vi "Unpack Control Drag Source Update.vi"(0 "ControlDragSourceUpdateMsg In":refnum<class "ControlDragSourceUpdateMsg.lvclass">) -> (4 "Ctl Refnum":refnum<vi>, 6 "Control Label":string, 8 "Time":u32, 10 "Result":enum16{"Drop Cancel", "Drop Move", "Drop Copy"}(ring))   [LabVIEW 2017, in "ActorEvents.lvlib" / "ControlDragSourceUpdateMsg.lvclass"]
doc: "<License>\nCopyright © 2017 Composed Systems, LLC | All rights reserved\nwww.composed.io\n\nAuthor: Ethan Stern <ethan.stern@composed.io>\n\nThis software is provided \"AS IS\" WITHOUT WARRANTIES, either express or implied, AND IS FOR EDUCATIONAL PURPOSES ONLY.\n</License>"
uses:
  ControlDragSourceUpdateMsg.lvclass
  ControlDragSourceUpdateMsg.lvclass/ControlDragSourceUpdateMsg.ctl
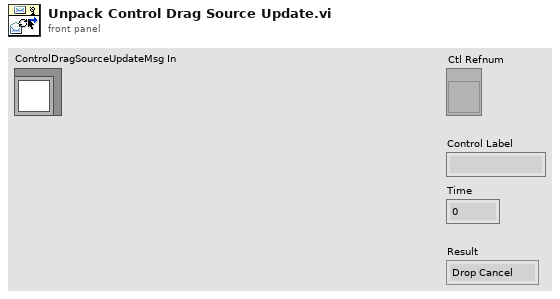
[diagram p1: front panel]
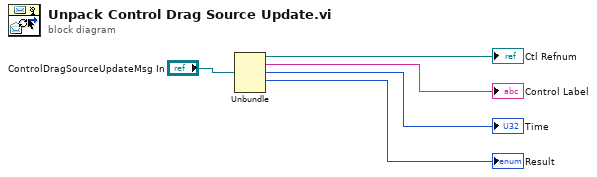
[diagram p0: block diagram]
diagram:
  n1 = Unbundle("ControlDragSourceUpdateMsg In") -> (→"Ctl Refnum":refnum<vi>, →"Control Label":string, →"Time":u32, →"Result":enum16{"Drop Cancel", "Drop Move", "Drop Copy"})  [unwired: 1 out]
